vi "PolStart-C.vi"(3 "error in (no error)":errorcluster, 4 "Sync In? (F)":bool, 5 "VISA resource name":refnum<visa-resource-name>) -> (0 "error out":errorcluster, 2 "VISA resource name out":refnum<visa-resource-name>)   [LabVIEW 2012]
doc: "Starts Polhemus output.\n\nNormally, sends a 'C' command.\n\nIf Sync In is enabled, sends a 'y1' command. IMPORTANT: after this command is enabled the the Polhemus only accepts and reports commands after each sync pulse. Thus, if this mode is enabled accidentally without ability to send a pulse, the unit must be restarted."
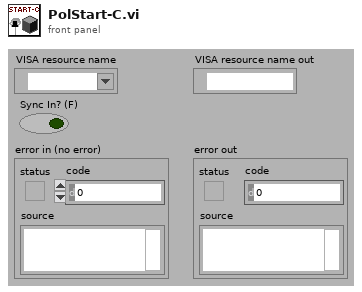
[diagram p1: front panel]
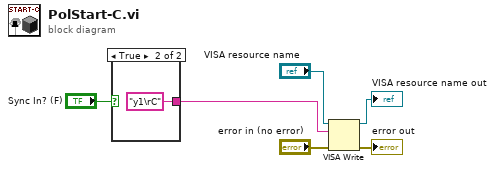
[diagram p0: block diagram]
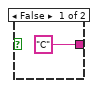
[diagram p2: hidden frame]
diagram:
  n1 = case shown="True" "Sync In? (F)" {
    tunnel: ["C" ("write buffer") "y1\rC" ("write buffer")] -> w4
    frame False {
    }
    frame True {
    }
  }
  n2 = VISA Write(VISA resource name="VISA resource name", write buffer=w4, error in (no error)="error in (no error)") -> (VISA resource name out=→"VISA resource name out":refnum<visa-resource-name>, error out=→"error out":errorcluster)  [unwired: 1 out]
